vi "Process.vi"(8 "error in (no error)":errorcluster, 10 "Pound in":refnum<class "Pound.lvclass">, 11 "Qbus in":refnum<class "Qbus.lvclass">) -> (0 "error out":errorcluster)   [LabVIEW 2017, in "McsaTestPanel.lvlib"]
doc: "Transfers real-time data to the Test Panel service on NI InsightCM Server. If your users do not require Test Panel support, you can omit this process from your device software."
uses:
  <vilib>/addons/InsightCM/Devices/Shared/Mcsa/McsaTestPanel/McsaTestPanel.lvlib
  <vilib>/addons/Qbus/Qbus.lvclass
  <vilib>/NI/Software Watchdog/Pound/Pound.lvclass
  <vilib>/addons/InsightCM/Devices/Shared/Mcsa/McsaTestPanel/controls/Configuration.ctl
  <vilib>/addons/InsightCM/Devices/Shared/Common/TestPanel/controls/Configuration.ctl
  <vilib>/addons/InsightCM/Devices/Shared/Common/TestPanel/controls/State.ctl
  <vilib>/addons/InsightCM/MessageBus/Base/controls/IRoutingSource.ctl
  <vilib>/addons/InsightCM/Devices/Shared/Mcsa/McsaTestPanel/controls/ChannelStatus.ctl
  <vilib>/addons/InsightCM/MessageBus/Base/controls/KeyValuePair.ctl
  <vilib>/NI/Software Watchdog/Watchdog/Watchdog.lvclass
  <vilib>/addons/InsightCM/Devices/Shared/Common/TestPanel/TestPanel.lvlib
  <vilib>/addons/InsightCM/Devices/Shared/Common/DataFlow/DataFlow.lvlib
  <vilib>/addons/InsightCM/Utilities/GlobalConfiguration/GlobalConfiguration.lvlib
  <vilib>/addons/InsightCM/Devices/Shared/Common/ServerComm/ServerComm.lvlib
  <vilib>/addons/TraceLogger/TraceLogger.lvlib
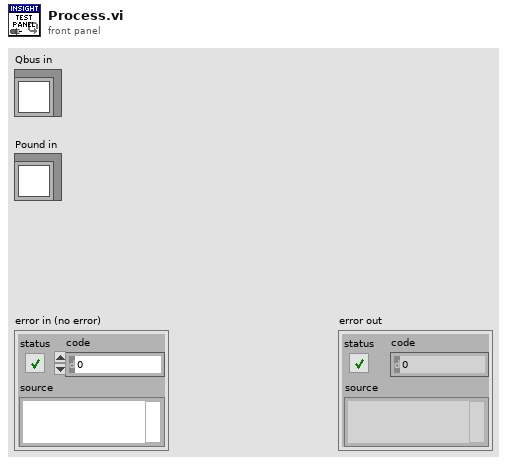
[diagram p1: front panel]
types:
  T1 = typedef "McsaTestPanel.lvlib/ChannelStatus.ctl" = cluster{"DataGroup":string, "ChannelStatus":T2[]}
  T2 = typedef "KeyValuePair.ctl" = cluster{"Key":string, "Value":string}
  T3 = typedef "McsaTestPanel.lvlib/Configuration.ctl" = cluster{"Common":T4, "ChanNameMap":variant}
  T4 = typedef "TestPanel.lvlib/Configuration.ctl" = cluster{"State":T5, "Waveform Channel":string, "DataGroup":string, "Number of Samples":i32, "Timeout":dbl, "History":variant, "LastRequest":timestamp, "BufferSize":i32, "OpState":variant, "IRoutingSource":T6}
  T5 = typedef "TestPanel.lvlib/State.ctl" = enum16{"Off", "On", "PendingValues", "PendingDataSet"}
  T6 = typedef "IRoutingSource.ctl" = cluster{"CorrelationId":string, "ReplyTo":string}
  T7 = typedef "DataFlow.lvlib/Data.ctl" = cluster{"DataGroup":string, "Waveforms":T8, "Map":T9, "Type":T10}
  T8 = typedef "wfmSGL_DVR.ctl" = refnum<data-value>
  T9 = typedef "PointValueMap.lvlib/PointMap.ctl" = refnum<data-value>
  T10 = typedef "DataFlow.lvlib/Type.ctl" = enum16{"High Rate", "Low Rate", "Burst Mode"}
  T11 = typedef "Message.ctl" = cluster{"Header":T12, "Body":u8[]}
  T12 = typedef "MessageHeader.ctl" = cluster{"MessageName":string, "Timestamp":i64, "CorrelationId":string, "ContentType":string, "RoutingKey":string, "Properties":T2[]}
  T13 = typedef "DeviceTestPanelGetTimeSeriesRequestBody.ctl" = cluster{"DataGroup":string, "TrendPointIds":string[]}
  T14 = typedef "DeviceTestPanelGetDataSetForChannelRequestBody.ctl" = cluster{"DataGroup":string, "ChannelName":string, "Properties":T2[]}
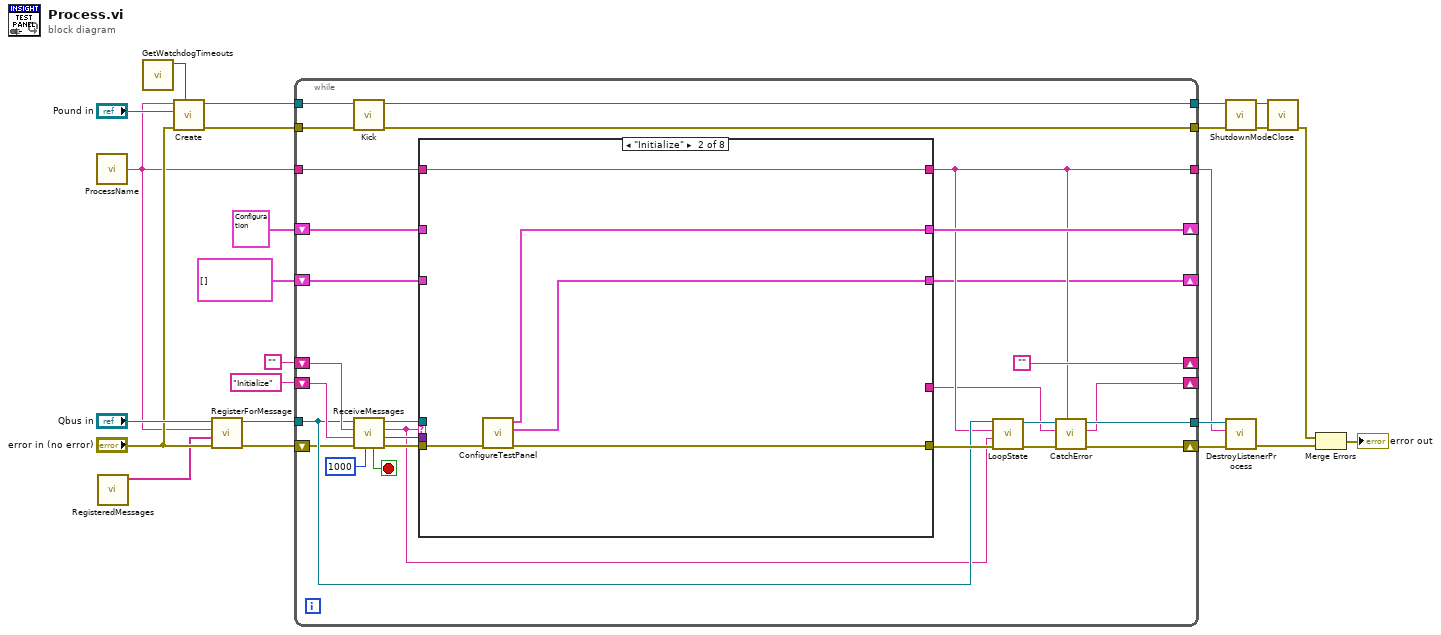
[diagram p0: block diagram]
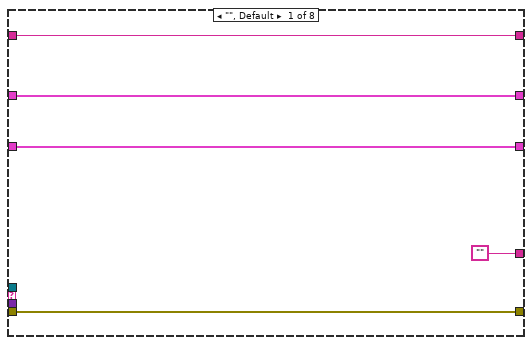
[diagram p2: hidden frame]
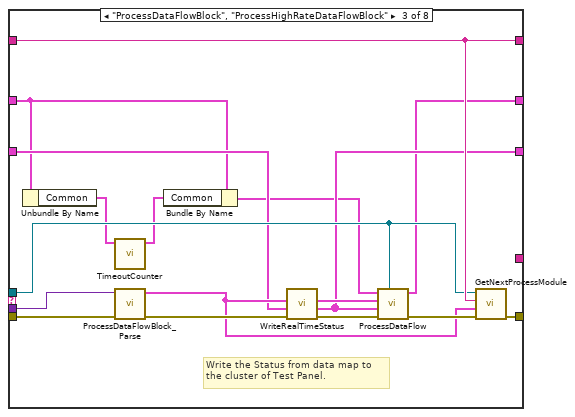
[diagram p3: hidden frame]
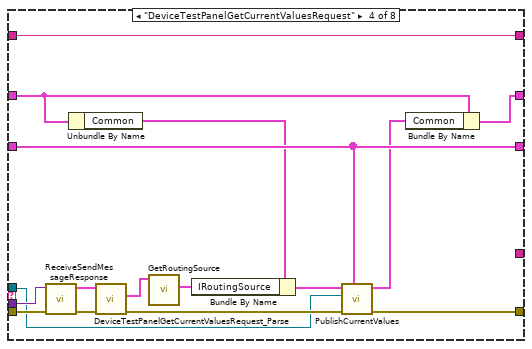
[diagram p4: hidden frame]
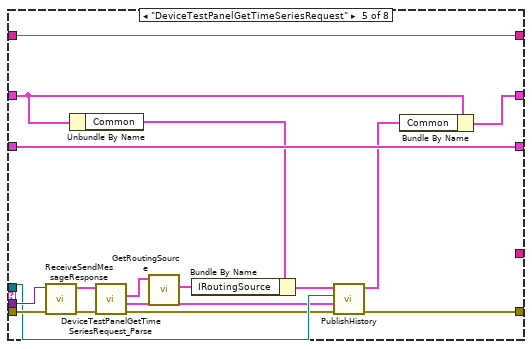
[diagram p5: hidden frame]
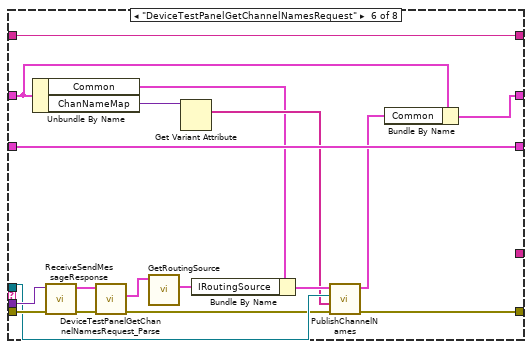
[diagram p6: hidden frame]
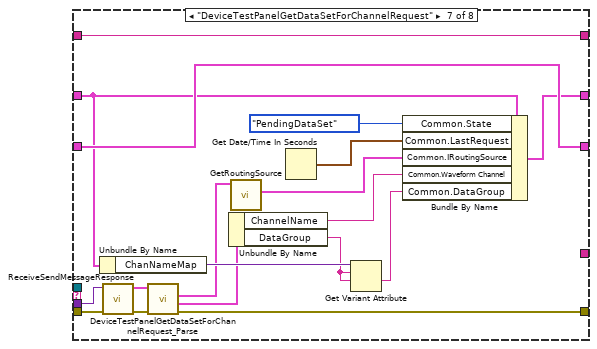
[diagram p7: hidden frame]
diagram:
  n1 = call <vilib>:"ProcessName.vi"() -> ("process name"=w1:string)  [unwired: 5 in]
  n2 = call <vilib>:"RegisteredMessages.vi"() -> ("registered messages"=w4:string[])  [unwired: 11 in]
  n3 = call <vilib>:"GetWatchdogTimeouts.vi"() -> ("software timeout"=w3:u32)  [unwired: 10 in, 1 out]
  n4 = call <vilib>:"Create.vi"("Execution Timeout (ms)"=w3, "error in (no error)"="error in (no error)", "Pound"="Pound in", "Name"=w1) -> ("error out"=w13:errorcluster, "Watchdog"=w18:refnum<data-value>)  [unwired: 6 in]
  n5 = call <vilib>:"RegisterForMessage.vi"("error in (no error)"="error in (no error)", "message names"=w4, "process name"=w1, "Qbus in"="Qbus in") -> ("error in (no error)"=w5:errorcluster, "Qbus out"=w7:refnum<class "Qbus.lvclass">)  [unwired: 6 in]
  n6 = while {
    shift-right: [""] -> _
    shift-left: "" -> [w51]
    tunnel: w7 -> [w39]
    tunnel: w1 -> [w29]
    tunnel: [w42] -> w22
    tunnel: [w28] -> w21
    shift-right: [w41] -> _
    shift-left: "Initialize" -> [w46]
    shift-right: [w44] -> _
    shift-left: T3 {"Common"={"State"=enum."Off", "Waveform Channel"="", "DataGroup"="", "Number of Samples"=0, "Timeout"=0.0, "History"=variant, "LastRequest"=timestamp(0 s since 1904-01-01), "BufferSize"=0, "OpState"=variant, "IRoutingSource"={"CorrelationId"="", "ReplyTo"=""}}, "ChanNameMap"=variant} ("Test Panel Config") -> [w45]
    tunnel: w18 -> [w38]
    tunnel: [w37] -> w15
    tunnel: w13 -> [w36]
    tunnel: [w34] -> w12
    shift-right: [w43] -> w23
    shift-left: w5 -> [w35]
    shift-right: [w26] -> _
    shift-left: T1[] [] ("DataGroups ChannelStatus") -> [w25]
    stop <- w52 stop-if-true
    n7 = call <vilib>:"Kick.vi"("error in (no error)"=w36, "Watchdog"=w38) -> ("error out"=w34:errorcluster, "Watchdog"=w37:refnum<data-value>)  [unwired: 8 in]
    n8 = call <vilib>:"ReceiveMessages.vi"("Timeout(1000)"=1000 ("milliseconds to wait"), "error in (no error)"=w35, "priority action"=w46, "default action"=w51, "Qbus in"=w39) -> ("error out"=w50:errorcluster, "message value"=w47:variant, "action"=w33:string, "Qbus out"=w48:refnum<class "Qbus.lvclass">, "exit"=w52:bool)  [unwired: 2 in]
    n9 = case shown="\"Initialize\"" w33 {
      tunnel: w50 -> [w53 w62 w76 w94 w110 w128 w147 w152]
      tunnel: w48 -> [_ _ w74 w85 w104 w121 _ _]
      tunnel: [w53 w60 w78 w87 w101 w119 w133 w152] -> w40
      tunnel: w47 -> [_ _ w77 w93 w107 w127 w146 _]
      tunnel: w45 -> [w57 _ w65 w81 w97 w115 w132 w151]
      tunnel: [w57 w58 w63 w80 w98 w113 w131 w151] -> w44
      tunnel: [w56 w61 w75 w95 w112 w130 w148 w150] -> w28
      tunnel: w29 -> [w56 w61 w75 w95 w112 w130 w148 w150]
      tunnel: ["" _ _ _ _ _ _ _] -> w27
      tunnel: [w54 w59 w68 w84 w100 w126 w141 w149] -> w26
      tunnel: w25 -> [w54 _ w69 w84 w100 w126 w141 w149]
      frame "", Default {
      }
      frame "Initialize" {
        n10 = call <vilib>:"ConfigureTestPanel.vi"("error in (no error)"=w62) -> ("error out"=w60:errorcluster, "DataGroups ChannelStatus"=w59:T1[], "Test Panel Config out"=w58:T3)  [unwired: 8 in]
      }
      frame "ProcessDataFlowBlock", "ProcessHighRateDataFlowBlock" {
        # "Write the Status from data map to \nthe cluster of Test Panel."
        n11 = Unbundle By Name(w65) -> ("Common"=w66:T4)
        n12 = call <vilib>:"TimeoutCounter.vi"("config in"=w66) -> ("config out"=w64:T4)  [unwired: 10 in]
        n13 = call <vilib>:"ProcessDataFlowBlock_Parse.vi"("error in (no error)"=w76, "body"=w77) -> ("error out"=w73:errorcluster, "data"=w72:T7)  [unwired: 8 in]
        n14 = Bundle By Name(cluster=w65, "Common"=w64) -> (w67:T3)
        n15 = call <vilib>:"WriteRealTimeStatus.vi"("error in (no error)"=w73, "DataGroups ChannelStatus in"=w69, "data in"=w72) -> ("error out"=w70:errorcluster, "DataGroups ChannelStatus out"=w68:T1[], "data out"=w71:T7)  [unwired: 6 in]
        n16 = call <vilib>:"ProcessDataFlow.vi"("Qbus in"=w74, "error in (no error)"=w70, "DataGroups ChannelStatus"=w68, "Data"=w71, "config in"=w67) -> ("error out"=w79:errorcluster, "config out"=w63:T3)  [unwired: 5 in]
        n17 = call <vilib>:"GetNextProcessModule.vi"("error in (no error)"=w79, "data"=w72, "source"=w75, "Qbus in"=w74) -> ("error out"=w78:errorcluster)  [unwired: 6 in, 1 out]
      }
      frame "DeviceTestPanelGetCurrentValuesRequest" {
        n18 = call <vilib>:"ReceiveSendMessageResponse.vi"("error in (no error)"=w94, "body"=w93) -> ("error out"=w92:errorcluster, "message"=w91:T11)  [unwired: 6 in, 2 out]
        n19 = Unbundle By Name(w81) -> ("Common"=w83:T4)
        n20 = call <vilib>:"DeviceTestPanelGetCurrentValuesRequest_Parse.vi"("error in (no error)"=w92, "Message"=w91) -> ("error out"=w88:errorcluster, "Header"=w90:T12)  [unwired: 7 in, 1 out]
        n21 = call <vilib>:"GetRoutingSource.vi"("Header in"=w90) -> ("IRoutingSource"=w89:T6)  [unwired: 9 in, 1 out]
        n22 = Bundle By Name(cluster=w83, "IRoutingSource"=w89) -> (w86:T4)
        n23 = call <vilib>:"PublishCurrentValues.vi"("DataGroups ChannelStatus"=w84, "error in (no error)"=w88, "Qbus in"=w85, "config in"=w86) -> ("error out"=w87:errorcluster, "config out"=w82:T4)  [unwired: 6 in]
        n24 = Bundle By Name(cluster=w81, "Common"=w82) -> (w80:T3)
      }
      frame "DeviceTestPanelGetTimeSeriesRequest" {
        n25 = call <vilib>:"ReceiveSendMessageResponse.vi"("error in (no error)"=w110, "body"=w107) -> ("error out"=w109:errorcluster, "message"=w108:T11)  [unwired: 6 in, 2 out]
        n26 = Unbundle By Name(w97) -> ("Common"=w99:T4)
        n27 = call <vilib>:"DeviceTestPanelGetTimeSeriesRequest_Parse.vi"("error in (no error)"=w109, "Message"=w108) -> ("error out"=w102:errorcluster, "Body"=w103:T13, "Header"=w106:T12)  [unwired: 6 in, 1 out]
        n28 = call <vilib>:"GetRoutingSource.vi"("Header in"=w106) -> ("IRoutingSource"=w111:T6)  [unwired: 9 in, 1 out]
        n29 = Bundle By Name(cluster=w99, "IRoutingSource"=w111) -> (w105:T4)
        n30 = call <vilib>:"PublishHistory.vi"("error in (no error)"=w102, "Body"=w103, "Qbus in"=w104, "config in"=w105) -> ("error out"=w101:errorcluster, "config out"=w96:T4)  [unwired: 6 in]
        n31 = Bundle By Name(cluster=w97, "Common"=w96) -> (w98:T3)
      }
      frame "DeviceTestPanelGetChannelNamesRequest" {
        n32 = Unbundle By Name(w115) -> ("Common"=w116:T4, "ChanNameMap"=w118:variant)
        n33 = call <vilib>:"ReceiveSendMessageResponse.vi"("error in (no error)"=w128, "body"=w127) -> ("error out"=w124:errorcluster, "message"=w125:T11)  [unwired: 6 in, 2 out]
        n34 = call <vilib>:"DeviceTestPanelGetChannelNamesRequest_Parse.vi"("error in (no error)"=w124, "Message"=w125) -> ("error out"=w120:errorcluster, "Header"=w123:T12)  [unwired: 7 in, 1 out]
        n35 = call <vilib>:"GetRoutingSource.vi"("Header in"=w123) -> ("IRoutingSource"=w129:T6)  [unwired: 9 in, 1 out]
        n36 = Get Variant Attribute(Variant=w118) -> (names=w117:string[])  [unwired: 3 in, 3 out]
        n37 = Bundle By Name(cluster=w116, "IRoutingSource"=w129) -> (w122:T4)
        n38 = call <vilib>:"PublishChannelNames.vi"("error in (no error)"=w120, "names"=w117, "Qbus in"=w121, "config in"=w122) -> ("error out"=w119:errorcluster, "config out"=w114:T4)  [unwired: 6 in]
        n39 = Bundle By Name(cluster=w115, "Common"=w114) -> (w113:T3)
      }
      frame "DeviceTestPanelGetDataSetForChannelRequest" {
        n40 = Unbundle By Name(w132) -> ("ChanNameMap"=w140:variant)
        n41 = call <vilib>:"ReceiveSendMessageResponse.vi"("error in (no error)"=w147, "body"=w146) -> ("error out"=w137:errorcluster, "message"=w136:T11)  [unwired: 6 in, 2 out]
        n42 = call <vilib>:"DeviceTestPanelGetDataSetForChannelRequest_Parse.vi"("error in (no error)"=w137, "Message"=w136) -> ("error out"=w133:errorcluster, "Body"=w135:T14, "Header"=w134:T12)  [unwired: 6 in, 1 out]
        n43 = Unbundle By Name(w135) -> ("ChannelName"=w145:string, "DataGroup"=w139:string)
        n44 = call <vilib>:"GetRoutingSource.vi"("Header in"=w134) -> ("IRoutingSource"=w142:T6)  [unwired: 9 in, 1 out]
        n45 = Get Date/Time In Seconds() -> (seconds since 1Jan1904=w144:timestamp)
        n46 = Get Variant Attribute(Variant=w140, name=w139, default value (empty Variant)=w139) -> (value=w138:string)  [unwired: 1 in, 3 out]
        n47 = Bundle By Name(cluster=w132, "Common.State"=State."PendingDataSet" ("State"), "Common.LastRequest"=w144, "Common.IRoutingSource"=w142, "Common.Waveform Channel"=w145, "Common.DataGroup"=w138) -> (w131:T3)
      }
      frame "Exit" {
      }
    }
    n48 = call <vilib>:"LoopState.vi"("error in (no error)"=w40, "loop action"=w33, "process name"=w28, "Qbus in"=w39) -> ("error out"=w31:errorcluster, "Qbus out"=w30:refnum<class "Qbus.lvclass">)  [unwired: 6 in]
    n49 = call <vilib>:"CatchError.vi"("source"=w28, "error in (no error)"=w31, "next action in"=w27, "Qbus in"=w30) -> ("error out"=w43:errorcluster, "next action out"=w41:string, "Qbus out"=w42:refnum<class "Qbus.lvclass">)  [unwired: 5 in]
  }
  n50 = call <vilib>:"ShutdownMode.vi"("error in (no error)"=w12, "Watchdog"=w15) -> ("error out"=w14:errorcluster, "Watchdog"=w16:refnum<data-value>)  [unwired: 8 in]
  n51 = call <vilib>:"DestroyListenerProcess.vi"("error in (no error)"=w23, "process name"=w21, "Qbus in"=w22) -> ("error in (no error)"=w11:errorcluster)  [unwired: 7 in, 1 out]
  n52 = call <vilib>:"Close.vi"("error in (no error)"=w14, "Watchdog"=w16) -> ("error out"=w10:errorcluster)  [unwired: 9 in]
  n53 = Merge Errors(w10, w11) -> (→"error out":errorcluster)
